vi "Hello World.vi"() -> ()   [LabVIEW 2011]
uses:
  VIremote.llb/VIremoteFunction.ctl
panel:
  in  "stop":bool
  out "Address to be entered on iOS device":string
  # "Hello World"
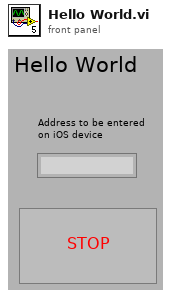
[diagram p1: front panel]
types:
  T1 = typedef "VIremoteFunction.ctl" = enum16{"Do nothing", "Stop controller", "Close this connection", "Show info panel", "Set VI to control", "Set Accelerometer freq (Hz)", "Show Alert message", "Start Sound Input", "Stop Sound Input", "Set Volume (0-100)", "Set sound output Speaker", "Set sound output Receiver", "Play Sound", "Repeat Sound", "Stop Sound", "Pause Sound", "Resume Sound", "Set panel width of caller (320 or 480)", "Set Panel Size to Portrait", "Set Panel Size to Landscape", "Set Panel Size as Current Orientation", "Allow all UI Orientations", "Send user notification", "Disable Scrolling", "Normal Scrolling", "Page Scrolling", "Set Scroll Offset", "Page Indicator Position"}
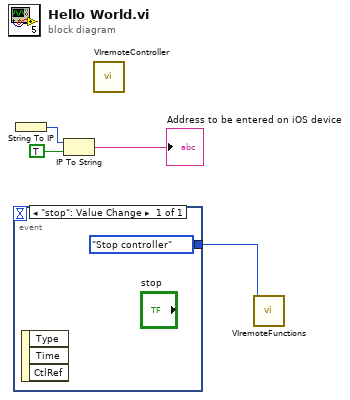
[diagram p0: block diagram]
diagram:
  n1 = event shown="[0] \"stop\": Value Change" {
    selector: _ -> [_]
    dyn-events: _ -> [_]
    timeout: _ -> [_]
    tunnel: [VIremoteFunction."Stop controller" ("Function")] -> w1
    event "stop": Value Change {
      n2 = event-data() -> ()  [unwired: 4 out]
    }
  }
  n3 = String To IP() -> (0:w4:u32)  [unwired: 1 out]
  n4 = IP To String(1:TRUE ("dot notation? (F)"), 2:w4) -> (0:→"Address to be entered on iOS device":string)
  n5 = call "VIremoteController.vi"() -> ()  [unwired: 1 in, 11 out]
  n6 = call "VIremoteFunctions.vi"("Function"=w1) -> ()  [unwired: 5 in, 6 out]
